vi "generate wvfrm.vi"(8 "error in (no error)":errorcluster) -> (0 "error out":errorcluster, 2 "waveform":dbl[](array[numeric]), 3 "time series":dbl[](array[numeric]), 4 "canceled?":bool)   [LabVIEW 2013]
doc: "Simulates a sine wave, square wave, triangle wave, sawtooth wave, or noise signal.\n--------------------\n\nThis Express VI is configured as follows:\n\nSignal Type: Sine\nFrequency: 10.1 Hz\nAmplitude: 1\nPhase: 0\nOffset: 0\nSampling Rate: 1000 Hz\nNumber of Samples: 100 (Automatic)\nTiming: Run as fast as possible\nTimestamps: Relative"
panel:
  in  "Cancel Button":bool
  in  "OK Button":bool
  in  "Generate":u16(ring) items=["Sine", "Square", "Triangle", "Sawtooth", "DC"]
  in  "Noise Type":u16(ring) items=["Uniform White Noise", "Gaussian White Noise", "Periodic Random Noise", "Gamma Noise", "Poisson Noise", "Binomial Noise", "Bernoulli Noise", "MLS Sequence "]
  in  "Add noise":bool
  in  "# of Samples":i32=100
  in  "Sampling Rate (Hz)":dbl=1000.0 format="%0.2f"
  in  "Seed Number":dbl=-1.0
  in  "Noise amplitude":dbl=0.6
  out "wvfrm":dynamicdata(graph) caption="Sine"
  in  "Duty Cycle (%)":dbl=50.0
  in  "Phase":dbl
  in  "Amplitude":dbl=1.0
  in  "Frequency":dbl=10.1
  in  "Offset":dbl
  # "Generate"
  # "Timing"
  # "Noise"
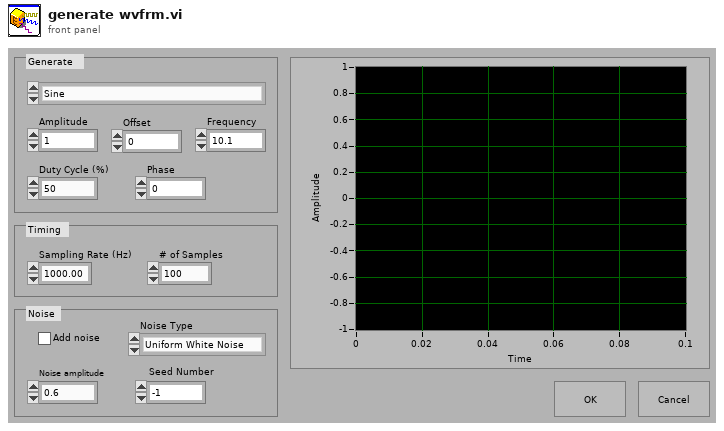
[diagram p1: front panel]
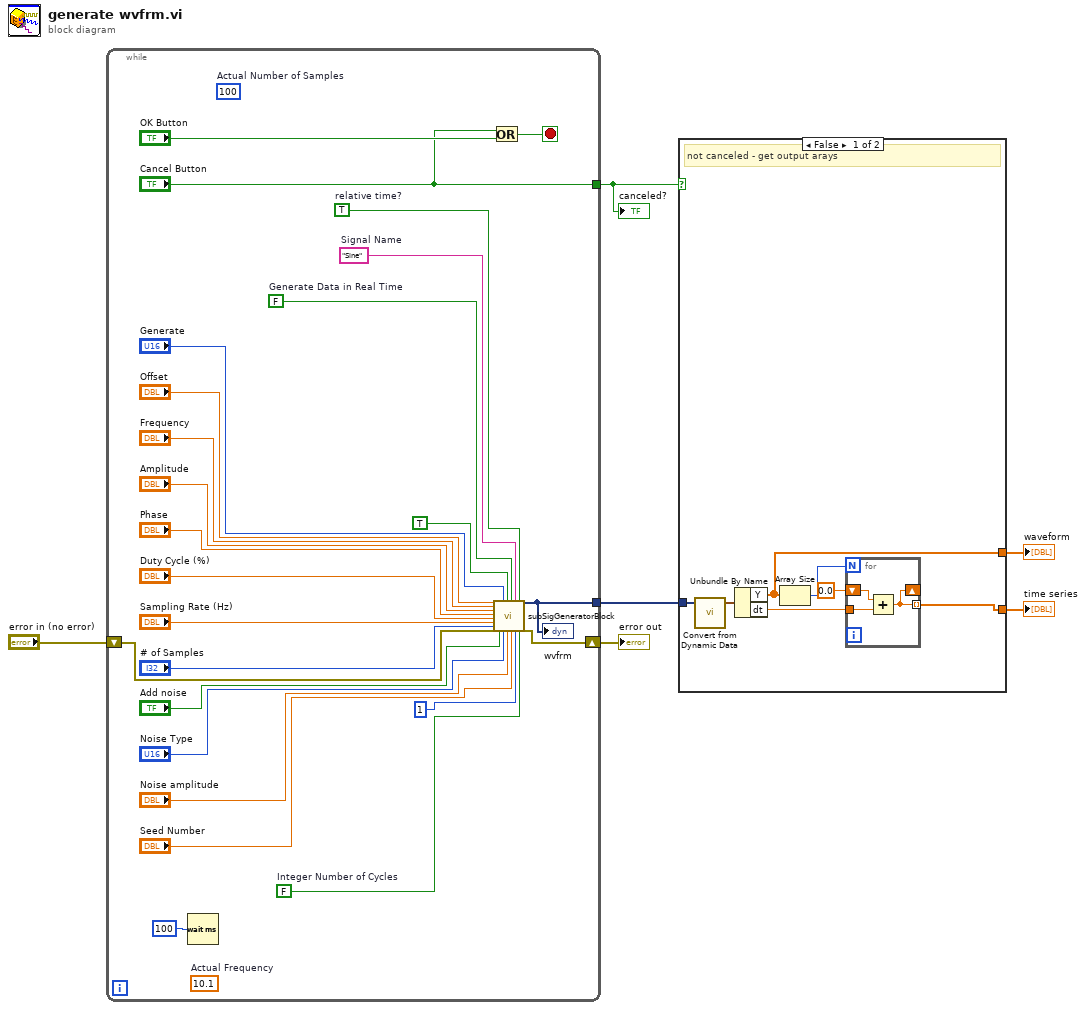
[diagram p0: block diagram]
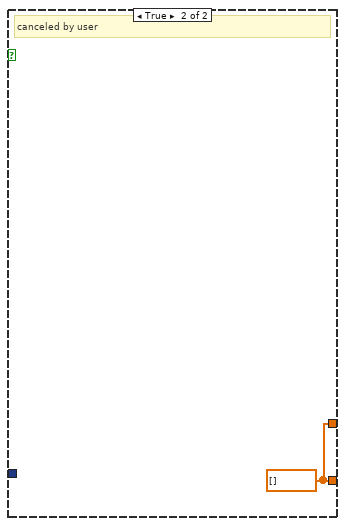
[diagram p2: hidden frame]
diagram:
  n1 = while {
    tunnel: ["Cancel Button"] -> w3
    shift-right: [w9] -> w6
    shift-left: "error in (no error)" -> [w8]
    tunnel: [w7] -> w4
    stop <- w11 stop-if-true
    (unwired) 10.1  # Actual Frequency
    (unwired) 100  # Actual Number of Samples
    w14 = FALSE  # Integer Number of Cycles
    w20 = TRUE  # relative time?
    w21 = "Sine"  # Signal Name
    w22 = FALSE  # Generate Data in Real Time
    n2 = Wait (ms)(milliseconds to wait=u32 100) -> ()  [unwired: 1 out]
    n3 = Or(x="Cancel Button", y="OK Button") -> (x .or. y?=w11:bool)
    n4 = call <vilib>:"subSigGeneratorBlock.vi"("Offset"="Offset", "Frequency"="Frequency", "Amplitude"="Amplitude", "Phase"="Phase", "Duty Cycle (%)"="Duty Cycle (%)", "Sampling Rate (Hz)"="Sampling Rate (Hz)", "# of Samples"="# of Samples", "error in (no error)"=w8, "Noise"="Add noise", "Generate"="Generate", "Noise Ring"="Noise Type", "Reset Signal"=TRUE, "Noise Amplitude"="Noise amplitude", "Generate Data in Real Time"=w22, "Seed Number"="Seed Number", "Signal Name"=w21, "trials"=1 ("Trials"), "relative time?"=w20, "Integer Number of Cycles"=w14) -> ("Signal"=w7:dynamicdata, "error out"=w9:errorcluster)  [unwired: 7 in]
    "wvfrm" <- w7
  }
  "canceled?" <- w3
  "error out" <- w6
  n5 = case shown="False" w3 {
    tunnel: w4 -> [w38 _]
    tunnel: [w33 w42] -> w2
    tunnel: [w32 w42] -> w1
    frame False {
      # "not canceled - get output arays"
      n6 = call "Convert from Dynamic Data"("Dynamic Data Type"=w38) -> ("Waveform"=w37:waveform(dbl))  [unwired: 3 in]
      n7 = Unbundle By Name(w37) -> ("Y"=w32:dbl[], "dt"=w35:dbl)
      n8 = Array Size(array=w32) -> (size(s)=w36:i32)
      n9 = for {
        N: w36 -> [_]
        tunnel: w35 -> [w41]
        shift-right: [w39] -> _
        shift-left: 0.0 ("dt") -> [w40]
        tunnel: [w39] -> w33 mode=indexing
        n10 = Add(x=w40, y=w41) -> (x+y=w39:dbl)
      }
    }
    frame True {
      w42 = dbl[] [] ("Y")
      # "canceled by user"
    }
  }
  "time series" <- w2
  "waveform" <- w1
